vi "ValueSignalByPathArray.vi"(0 "VI Reference In":refnum<vi>, 5 "Control Path":string[](array[string]), 7 "Value (Signaling)":variant, 11 "error in":errorcluster) -> (4 "VI Reference Out":refnum<vi>, 15 "error out":errorcluster)   [LabVIEW 2016]
doc: "This VI sets the value of controls in other VI. The control path is given as an array."
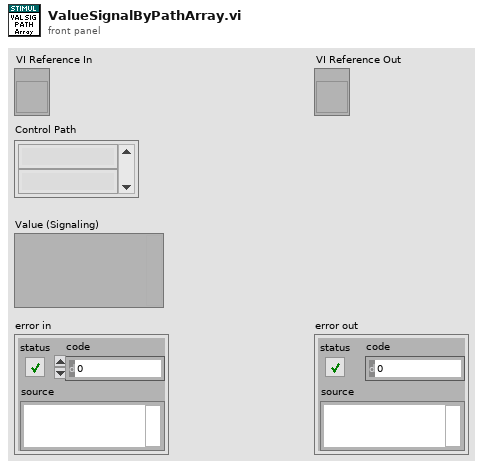
[diagram p1: front panel]
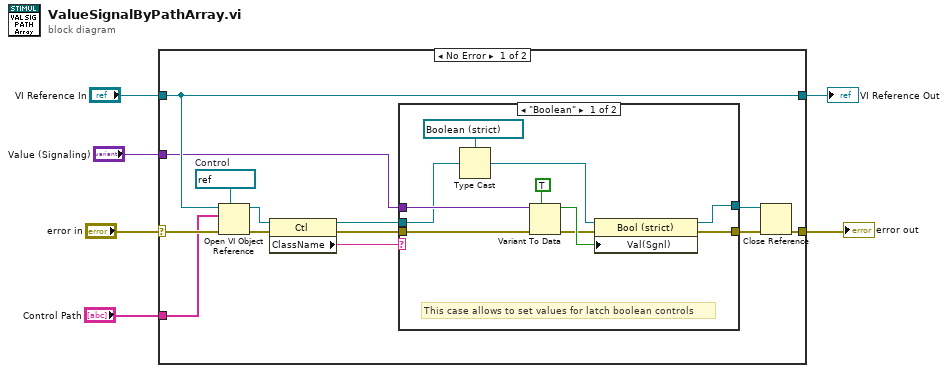
[diagram p0: block diagram]
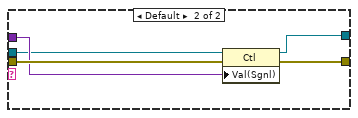
[diagram p2: hidden frame]
diagram:
  n1 = case shown="No Error" "error in" {
    selector: "error in" -> [w19 w36]
    tunnel: "Control Path" -> [w15 _]
    tunnel: "VI Reference In" -> [w18 w35]
    tunnel: [w18 w35] -> w3
    tunnel: "Value (Signaling)" -> [w10 _]
    tunnel: [w13 w36] -> w1
    frame No Error {
      w14 = refnum<vi> refnum  # Control
      n2 = Open VI Object Reference(7:w14, 8:w19, 10:w15, 11:w18) -> (0:w16:errorcluster, 3:w17:refnum<vi>)
      n3 = property class="Ctl"(reference=w17, error in=w16) -> (reference out=w7:refnum<vi>, error out=w12:errorcluster, "ClassName"=w11:string)
      n4 = case shown="\"Boolean\"" w11 {
        tunnel: [w27 w34] -> w9
        tunnel: [w28 w33] -> w8
        tunnel: w12 -> [w25 w32]
        tunnel: w10 -> [w23 w31]
        tunnel: w7 -> [w22 w30]
        frame "Boolean" {
          # "This case allows to set values for latch boolean controls"
          n5 = Type Cast(type=refnum<vi> refnum ("OK"), x=w22) -> (*(type *) &x=w29:refnum<vi>)
          n6 = Variant To Data(error in=w25, type=TRUE, Variant=w23) -> (data=w26:bool, error out=w24:errorcluster)
          n7 = property class="Bool (strict)"(reference=w29, error in=w24, "Val(Sgnl)"=w26) -> (reference out=w28:refnum<vi>, error out=w27:errorcluster)
        }
        frame Default {
          n8 = property class="Ctl"(reference=w30, error in=w32, "Val(Sgnl)"=w31) -> (reference out=w33:refnum<vi>, error out=w34:errorcluster)
        }
      }
      n9 = Close Reference(reference=w8, error in (no error)=w9) -> (error out=w13:errorcluster)
    }
    frame Error {
    }
  }
  "error out" <- w1
  "VI Reference Out" <- w3
